vi "emi_ Set Dialog Background.vi"(5 "VI Refnum(This vi)":refnum<vi>, 9 "error in (no error)":errorcluster) -> (6 "VI Refnum":refnum<vi>, 10 "error out":errorcluster)   [LabVIEW 2011]
doc: "Sets teh colors of teh Panel background to the dialog window system 01 color settings\nIf no VI ref in, then the VI containing this VI is used.\nIf VI has multiple panes, only the first pane will be used.\n\nOn error in: Does not run."
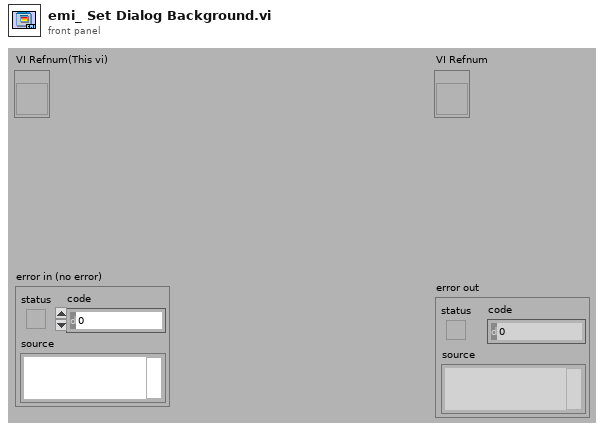
[diagram p1: front panel]
types:
  T1 = typedef "emi_System Colors.ctl" = cluster{"Main Top Panels":T2, "Main Botom Panels":T2, "Graphs":T2, "Dialogs":T2}
  T2 = typedef "_emi_ Color defenition.ctl" = cluster{"Type":T3, "Dark/Primary Color":u32, "Light/Secondary Color":u32, "Extra Color":u32}
  T3 = typedef "emi_List Of Graphix.ctl" = enum16{"FlatColor", "SharpGrad", "ShallowGrad", "GlasGradBord", "GlasGrad", "GlasGradBord 2"}
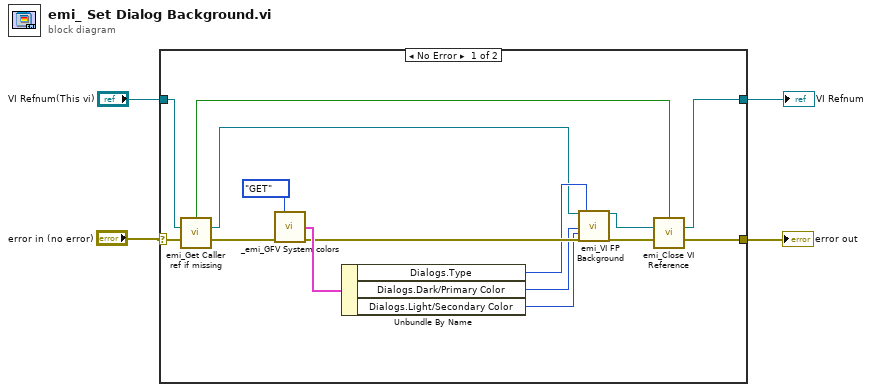
[diagram p0: block diagram]
diagram:
  n1 = case shown="No Error" "error in (no error)" {
    selector: "error in (no error)" -> [w18 w21]
    tunnel: [w16 w21] -> w4
    tunnel: "VI Refnum(This vi)" -> [w17 w20]
    tunnel: [w15 w20] -> w2
    frame No Error {
      n2 = call "emi_Get Caller ref if missing.vi"("VI Refnum(Calling VI)"=w17, "error in (no error)"=w18) -> ("Ref Generated"=w19:bool, "VI Refnum Out"=w8:refnum<vi>, "error out"=w12:errorcluster)  [unwired: 11 in]
      n3 = call "_emi_GFV System colors.vi"("Action(GET)"=enum16{"GET", "SET"}."GET", "error in (no error)"=w12) -> ("System background out"=w14:T1, "error out"=w11:errorcluster)  [unwired: 12 in]
      n4 = Unbundle By Name(w14) -> ("Dialogs.Type"=w9:T3, "Dialogs.Dark/Primary Color"=w6:u32, "Dialogs.Light/Secondary Color"=w5:u32)
      n5 = call "emi_VI FP Background.vi"("VI Refnum(This VI)"=w8, "Dark(Black)"=w6, "Light(White)"=w5, "error in"=w11, "Graphic Type(Flat Color)"=w9) -> ("VI Refnum out"=w7:refnum<vi>, "error IO"=w10:errorcluster)  [unwired: 13 in]
      n6 = call "emi_Close VI Reference.vi"("Close ref?(T)"=w19, "VI Refnum"=w7, "error in (no error)"=w10) -> ("VI Refnum Out"=w15:refnum<vi>, "error out"=w16:errorcluster)  [unwired: 11 in]
    }
    frame Error {
    }
  }
  "error out" <- w4
  "VI Refnum" <- w2
